vi "Timer.vi"(0 "Timers_Start":bool[](array[boolean]), 2 "Wait_Time":dbl=10.0 format="%#_13g", 11 "Error_In":errorcluster, 13 "Timer_Select":T1=enum."Start_Timer") -> (4 "Timer_Time":dbl[](array[numeric]), 6 "Time_Out?":bool[](array[boolean]), 15 "Error_Out":errorcluster)   [LabVIEW 2021]
doc: "Used for time out opertion."
uses:
  Controls/Timer_Data.ctl
  Controls/Timer_Operation_Select.ctl
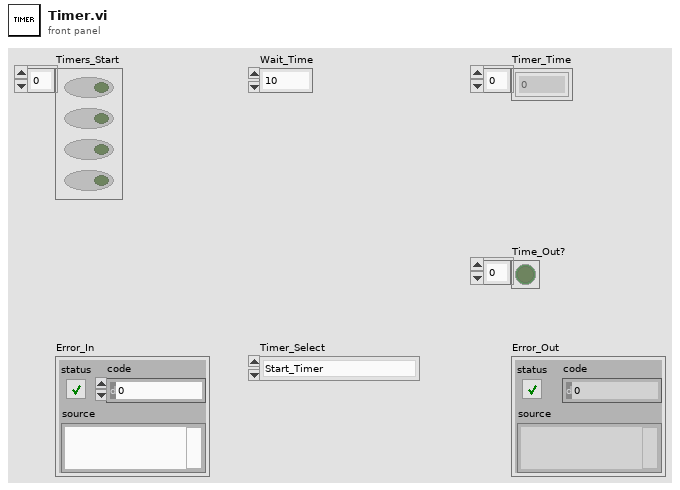
[diagram p1: front panel]
types:
  T1 = typedef "Timer_Operation_Select.ctl" = enum16{"Initialize", "Start_Timer", "Time_Out?", "Stop_Timer"}
  T2 = typedef "Timer_Data.ctl" = cluster{"T1_Start_Time":timestamp[], "T_Start?":bool[], "Wait_Time":dbl}
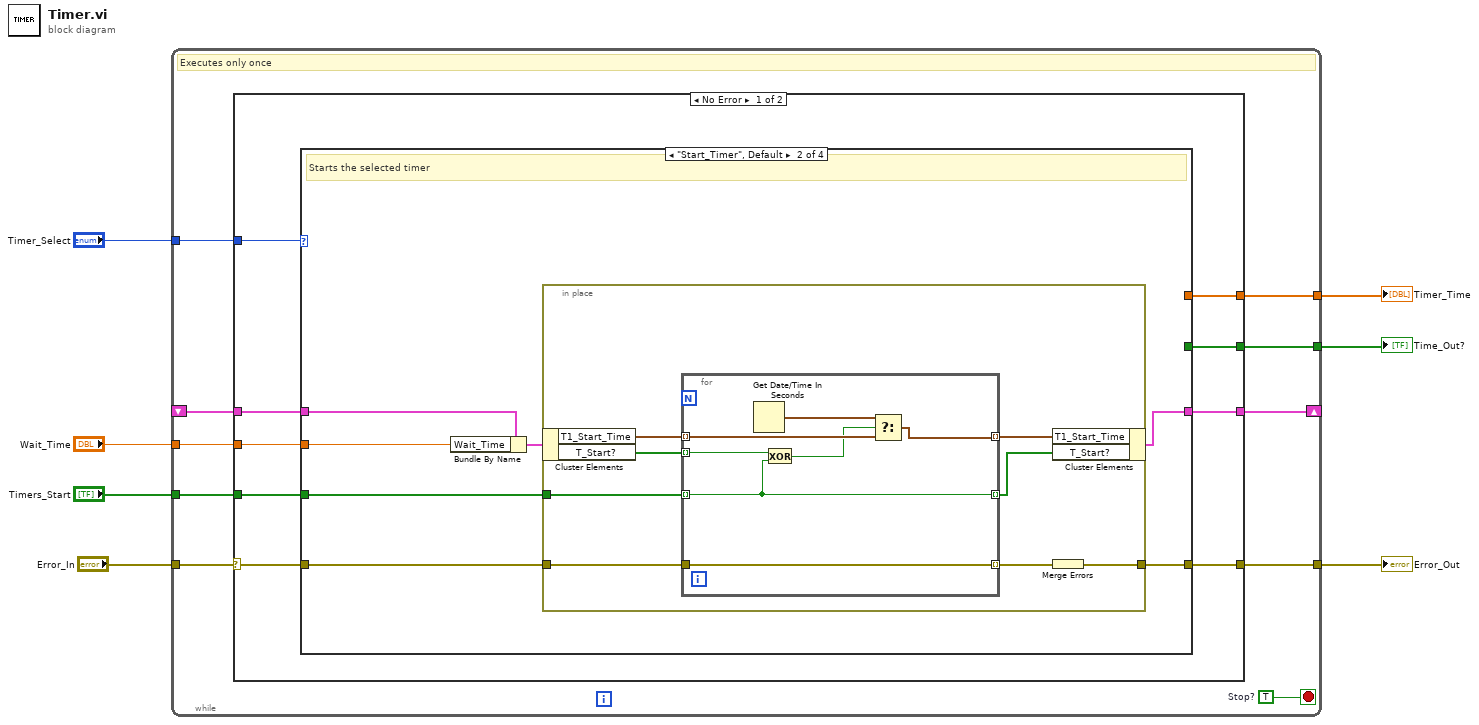
[diagram p0: block diagram]
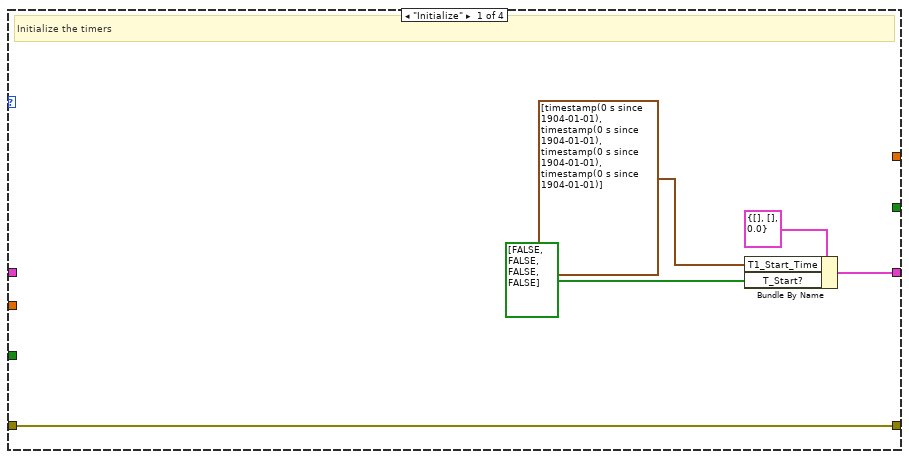
[diagram p2: hidden frame]
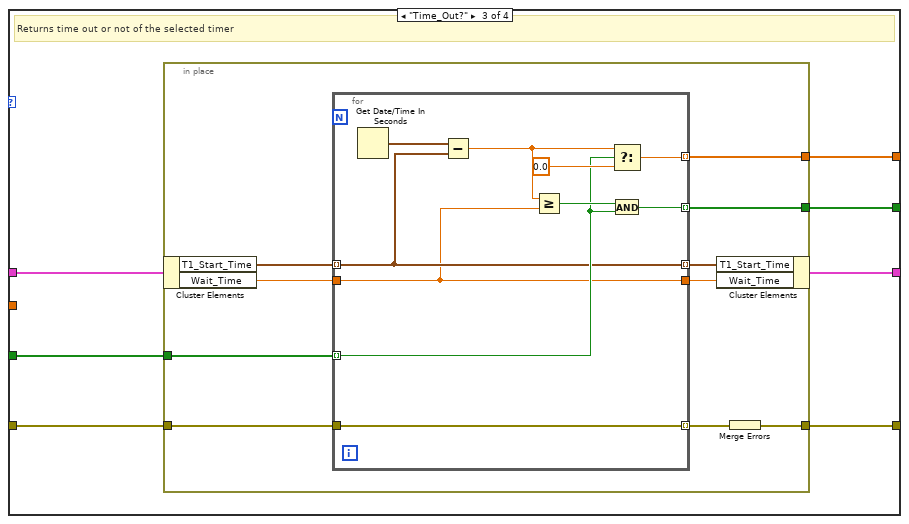
[diagram p3: hidden frame]
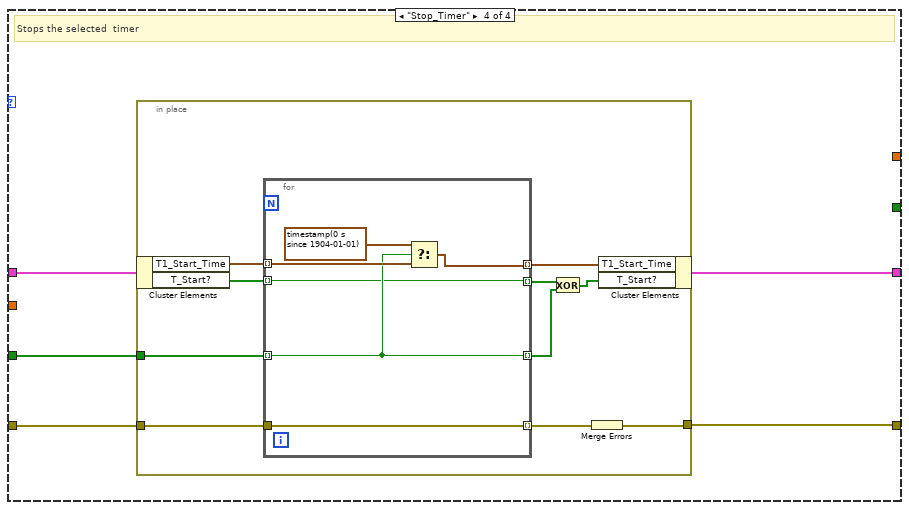
[diagram p4: hidden frame]
diagram:
  n1 = while {
    tunnel: "Error_In" -> [w16]
    tunnel: [w15] -> w6
    shift-right: [w12] -> _
    shift-left: _ -> [w14]
    tunnel: "Timer_Select" -> [w13]
    tunnel: "Wait_Time" -> [w11]
    tunnel: "Timers_Start" -> [w10]
    tunnel: [w9] -> w2
    tunnel: [w8] -> w1
    stop <- w17 stop-if-true
    w17 = TRUE  # Stop?
    # "Executes only once"
    n2 = case shown="No Error" w16 {
      selector: w16 -> [w26 w103]
      tunnel: [w25 w103] -> w15
      tunnel: w14 -> [w24 w102]
      tunnel: w13 -> [w22 _]
      tunnel: [w23 w102] -> w12
      tunnel: w11 -> [w21 _]
      tunnel: w10 -> [w20 _]
      tunnel: [w19 _] -> w9
      tunnel: [w18 _] -> w8
      frame No Error {
        n3 = case shown="\"Start_Timer\", Default" w22 {
          tunnel: w26 -> [w30 w38 w60 w81]
          tunnel: [w30 w37 w59 w82] -> w25
          tunnel: w24 -> [_ w34 w57 w84]
          tunnel: [w29 w36 w58 w85] -> w23
          tunnel: w21 -> [_ w35 _ _]
          tunnel: w20 -> [_ w32 w56 w83]
          tunnel: [_ _ w55 _] -> w19
          tunnel: [_ _ w54 _] -> w18
          frame "Initialize" {
            # "Initialize the timers"
            n4 = Bundle By Name(cluster=T2 {"T1_Start_Time"=[], "T_Start?"=[], "Wait_Time"=0.0}, "T1_Start_Time"=timestamp[] [timestamp(0 s since 1904-01-01), timestamp(0 s since 1904-01-01), timestamp(0 s since 1904-01-01), timestamp(0 s since 1904-01-01)], "T_Start?"=bool[] [FALSE, FALSE, FALSE, FALSE]) -> (w29:T2)
          }
          frame "Start_Timer", Default {
            # "Starts the selected timer"
            n5 = Bundle By Name(cluster=w34, "Wait_Time"=w35) -> (w33:T2)
            n6 = in-place {
              in-place-border: w38 -> [w42]
              in-place-border: [w41] -> w37
              in-place-border: w32 -> [w46]
              n7 = in-place-cluster #1(w33) -> ("T1_Start_Time"=w45:timestamp[], "T_Start?"=w40:bool[])
              n8 = for {
                tunnel: w46 -> [w48] mode=indexing
                tunnel: w45 -> [w52] mode=indexing
                tunnel: [w51] -> w44 mode=indexing
                tunnel: [w50] -> w43 mode=indexing
                tunnel: w42 -> [w50]
                tunnel: w40 -> [w49] mode=indexing
                tunnel: [w48] -> w39 mode=indexing
                n9 = Get Date/Time In Seconds() -> (seconds since 1Jan1904=w53:timestamp)
                n10 = Exclusive Or(1:w48, 2:w49) -> (0:w47:bool)
                n11 = Select(t=w53, s=w47, f=w52) -> (s? t:f=w51:timestamp)
              }
              n12 = in-place-cluster #1("T1_Start_Time"=w44, "T_Start?"=w39) -> (w36:T2)
              n13 = Merge Errors(w43) -> (w41:errorcluster)
            }
          }
          frame "Time_Out?" {
            # "Returns time out or not of the selected timer"
            n14 = in-place {
              in-place-border: w60 -> [w63]
              in-place-border: [w61] -> w59
              in-place-border: [w70] -> w55
              in-place-border: [w69] -> w54
              in-place-border: w56 -> [w66]
              n15 = in-place-cluster #2(w57) -> ("T1_Start_Time"=w68:timestamp[], "Wait_Time"=w67:dbl)
              n16 = for {
                tunnel: [w80] -> w70 mode=indexing
                tunnel: [w77] -> w69 mode=indexing
                tunnel: w68 -> [w73] mode=indexing
                tunnel: w67 -> [w72]
                tunnel: w66 -> [w74] mode=indexing
                tunnel: [w73] -> w65 mode=indexing
                tunnel: [w72] -> w64
                tunnel: w63 -> [w71]
                tunnel: [w71] -> w62 mode=indexing
                n17 = Get Date/Time In Seconds() -> (seconds since 1Jan1904=w79:timestamp)
                n18 = Subtract(x=w79, y=w73) -> (x-y=w78:dbl)
                n19 = Greater Or Equal?(x=w78, y=w72) -> (x >= y?=w75:bool)
                n20 = Select(t=w78, s=w74, f=0.0) -> (s? t:f=w77:dbl)
                n21 = And(x=w75, y=w74) -> (x .and. y?=w80:bool)
              }
              n22 = in-place-cluster #2("T1_Start_Time"=w65, "Wait_Time"=w64) -> (w58:T2)
              n23 = Merge Errors(w62) -> (w61:errorcluster)
            }
          }
          frame "Stop_Timer" {
            # "Stops the selected  timer"
            n24 = in-place {
              in-place-border: w83 -> [w93]
              in-place-border: [w90] -> w82
              in-place-border: w81 -> [w91]
              n25 = in-place-cluster #3(w84) -> ("T1_Start_Time"=w95:timestamp[], "T_Start?"=w89:bool[])
              n26 = for {
                tunnel: w95 -> [w100] mode=indexing
                tunnel: [w99] -> w94 mode=indexing
                tunnel: w93 -> [w97] mode=indexing
                tunnel: [w98] -> w92 mode=indexing
                tunnel: w91 -> [w98]
                tunnel: [w97] -> w87 mode=indexing
                tunnel: w89 -> [w96] mode=indexing
                tunnel: [w96] -> w88 mode=indexing
                n27 = Select(t=timestamp(0 s since 1904-01-01), s=w97, f=w100) -> (s? t:f=w99:timestamp)
              }
              n28 = Exclusive Or(1:w87, 2:w88) -> (0:w86:bool[])
              n29 = Merge Errors(w92) -> (w90:errorcluster)
              n30 = in-place-cluster #3("T1_Start_Time"=w94, "T_Start?"=w86) -> (w85:T2)
            }
          }
        }
      }
      frame Error {
      }
    }
  }
  "Error_Out" <- w6
  "Timer_Time" <- w1
  "Time_Out?" <- w2
